vi "dvp Vi Get Manufacturer.vi"(9 "nLength":u32, 10 "Manufacturer":string, 11 "handle":u32) -> (2 "Manufacturer out":string, 3 "function return":u32(ring))   [LabVIEW 2018, in "LabViewDVPCamera.lvlib"]
doc: "LabviewDvp2Api dvpStatus dvpViGetManufacturer(dvpHandle handle, char *Manufacturer, dvpUint32 nLength);"
uses:
  LabViewDVPCamera.lvlib
  LabViewDVPCamera/LabViewDVPCamera.dll
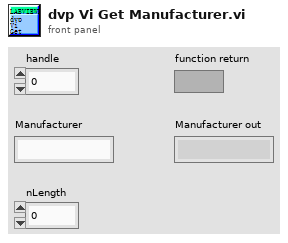
[diagram p1: front panel]
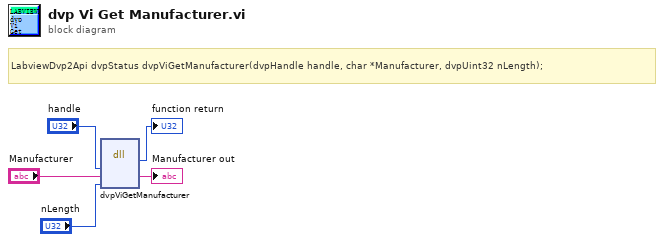
[diagram p0: block diagram]
diagram:
  # "LabviewDvp2Api dvpStatus dvpViGetManufacturer(dvpHandle handle, char *Manufacturer, dvpUint32 nLength);"
  n1 = dll-call lib="C:/Program Files (x86)/DVP2 Labview cn 64/Sample/LabViewDVPCamera/LabViewDVPCamera.*" fn="dvpViGetManufacturer"("handle"="handle", "Manufacturer"="Manufacturer", "nLength"="nLength") -> (→"function return":u32, "Manufacturer"=→"Manufacturer out":string)  [unwired: 5 in, 2 out]
